vi "Forward Message.vi"(6 "priority":i32, 8 "error in (no error)":errorcluster, 9 "Message in":refnum<class "Message.lvclass">, 10 "Target Enq":refnum<class "Message Enqueuer.lvclass">, 11 "Proxy in":refnum<class "Proxy.lvclass">) -> (0 "error out":errorcluster, 3 "Proxy out":refnum<class "Proxy.lvclass">)   [LabVIEW 2014, in "Proxy.lvlib" / "Proxy.lvclass"]
uses:
  Proxy.lvclass
  <vilib>/ActorFramework/Message/Message.lvclass
  <vilib>/ActorFramework/Message Enqueuer/Message Enqueuer.lvclass
  <vilib>/ActorFramework/Message Enqueuer/Message Enqueuer.lvclass/Message Enqueuer.ctl
  <vilib>/ActorFramework/Message Priority Queue/Priority Enqueue.vi
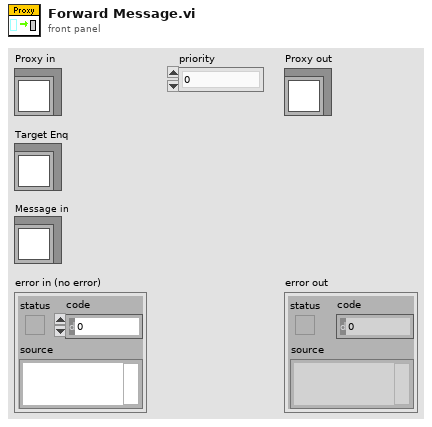
[diagram p1: front panel]
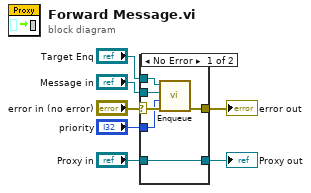
[diagram p0: block diagram]
diagram:
  n1 = case shown="No Error" "error in (no error)" {
    selector: "error in (no error)" -> [w12 w15]
    tunnel: [w11 w15] -> w6
    tunnel: [w13 w14] -> w4
    tunnel: "Proxy in" -> [w13 w14]
    tunnel: "Target Enq" -> [w10 _]
    tunnel: "Message in" -> [w9 _]
    tunnel: "priority" -> [w8 _]
    frame No Error {
      n2 = call <vilib>:"Enqueue.vi"("error in (no error)"=w12, "Message Priority (Normal)"=w8, "Message"=w9, "Message Enqueuer in"=w10) -> ("error out"=w11:errorcluster)  [unwired: 6 in, 1 out]
    }
    frame Error {
    }
  }
  "error out" <- w6
  "Proxy out" <- w4
